vi "ControlArmInterfaceEthernet.vi"() -> ()   [LabVIEW 2024]
panel:
  in  "stop":bool
  out "value":T1
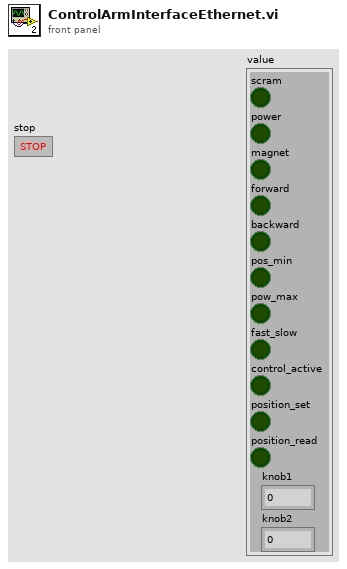
[diagram p1: front panel]
types:
  T1 = cluster{"scram":bool, "power":bool, "magnet":bool, "forward":bool, "backward":bool, "pos_min":bool, "pow_max":bool, "fast_slow":bool, "control_active":bool, "position_set":bool, "position_read":bool, "knob1":dbl, "knob2":dbl}
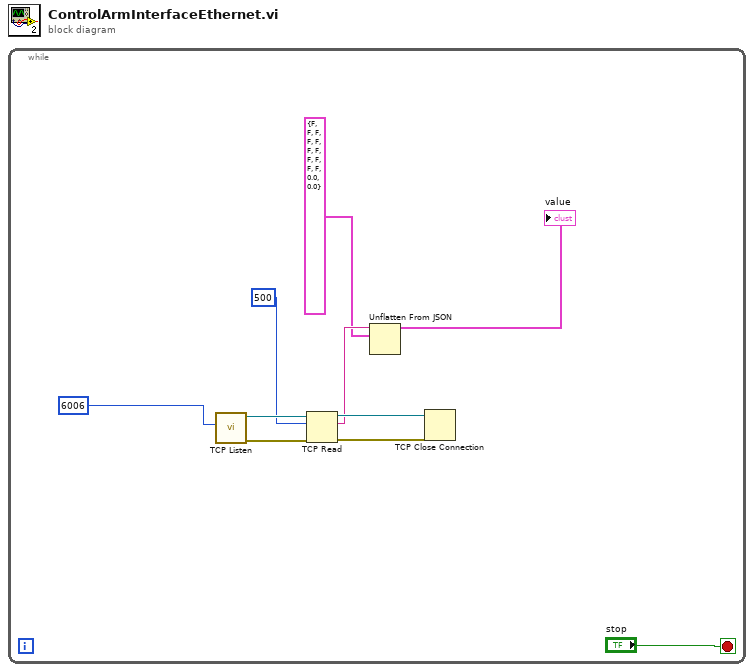
[diagram p0: block diagram]
diagram:
  n1 = while {
    stop <- "stop" stop-if-true
    n2 = call <vilib>:"TCP Listen.vi"("port"=u16 6006) -> ("error out"=w8:errorcluster, "connection ID"=w9:refnum<k5>)  [unwired: 6 in, 3 out]
    n3 = TCP Read(connection ID=w9, bytes to read=500, error in (no error)=w8) -> (connection ID out=w6:refnum<k5>, data out=w4:string, error out=w5:errorcluster)  [unwired: 2 in]
    n4 = Unflatten From JSON(JSON string=w4, type and defaults=T1 {"scram"=FALSE, "power"=FALSE, "magnet"=FALSE, "forward"=FALSE, "backward"=FALSE, "pos_min"=FALSE, "pow_max"=FALSE, "fast_slow"=FALSE, "control_active"=FALSE, "position_set"=FALSE, "position_read"=FALSE, "knob1"=0.0, "knob2"=0.0} ("Cluster")) -> (value=→"value":T1)  [unwired: 5 in, 1 out]
    n5 = TCP Close Connection(connection ID=w6, error in (no error)=w5) -> ()  [unwired: 1 in, 2 out]
  }
